vi "Main.vi"(8 "error in":errorcluster, 11 "Acq Cam Basler in":refnum<class "Acq Cam Basler.lvclass">) -> (0 "error out":errorcluster, 3 "Acq Cam Basler out":refnum<class "Acq Cam Basler.lvclass">)   [LabVIEW 2023, in "Acq Cam Basler.lvclass"]
doc: "The Queued Message Handler of a Worker."
uses:
  Acq Cam Basler.lvclass
  C:/Program Files (x86)/National Instruments/LabVIEW 2023/vi.lib/addons/_Workers/Library/Classes/Worker/Worker.lvclass
  Initialization Data.ctl
  UI Cam Basler/Parsed Data Acquisition.ctl
  UI Cam Basler/Data Image.ctl
  <vilib>/vision/Image Controls.llb/IMAQ Image.ctl
  <vilib>/addons/_Workers/Library/Classes/Message Queue/Message Queue.lvclass
  Etat Acquisition.ctl
  <vilib>/userDefined/High Color/IMAQdx.ctl
  Acq Cam Basler.lvclass/Acq Cam Basler.ctl
  <vilib>/addons/_Workers/Library/Classes/Message/Enqueue Message to Self v2 - Silent Mode.vi
  <vilib>/addons/_Workers/Library/Classes/Message/Message.lvclass
  <vilib>/vision/driver/NI_Vision_Acquisition_Software.lvlib
  UI Cam Basler/UI Cam Basler.lvclass
  C:/Program Files (x86)/National Instruments/LabVIEW 2023/vi.lib/addons/_Workers/Library/Classes/Workers Object/Workers Object.lvclass
  C:/Users/flepetit/Desktop/CamView-mdi-LV/Workers/Acq Cam Basler/Acq Cam Basler.lvclass
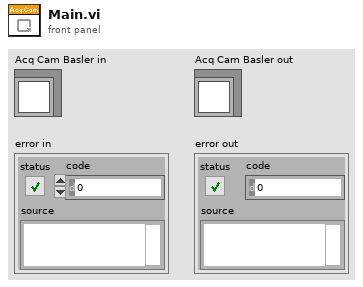
[diagram p1: front panel]
types:
  T1 = typedef "IMAQdx.ctl" = refnum<k21>
  T2 = typedef "Acq Cam Basler.lvclass/Etat Acquisition.ctl" = enum16{"Acquire", "Idle"}
  T3 = typedef "Acq Cam Basler.lvclass/Initialization Data.ctl" = cluster{"String":string, "Parsed Data Acquisition":T4, "Data Display":refnum<notifier>, "UI Cam Queue":refnum<class "Message Queue.lvclass">}
  T4 = typedef "UI Cam Basler.lvclass/Parsed Data Acquisition.ctl" = cluster{"Config Acquisition":cluster{"Camera name":string, "Gain":dbl, "Shutter(us)":dbl, "ROI":bool, "ROI coor":T5, "Palette":u32, "ModelName":string, "Pos X Ch":u32, "Pos Y Ch":u32, "Crosshair":bool}}
  T5 = typedef "IMAQ Rectangle" = cluster{"Left":i32, "Top":i32, "Right":i32, "Bottom":i32, "Rotation":dbl}
  T6 = typedef "IMAQ Image.ctl" = refnum<image>
  T7 = typedef "Workers.lvlib/Case Label.ctl" = string
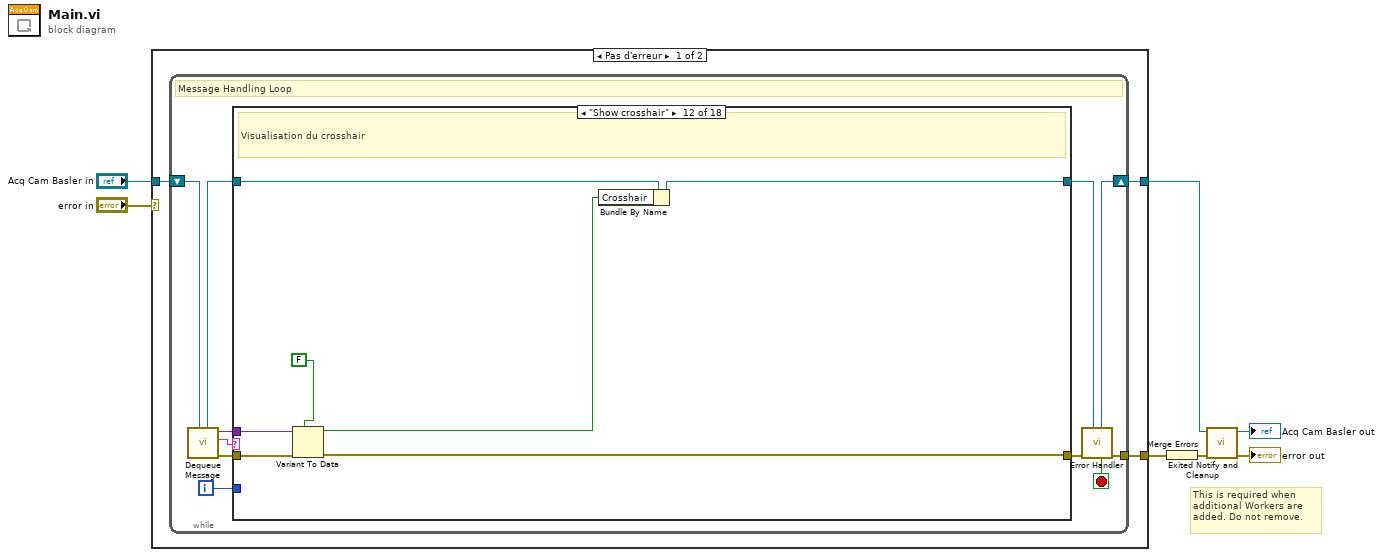
[diagram p0: block diagram]
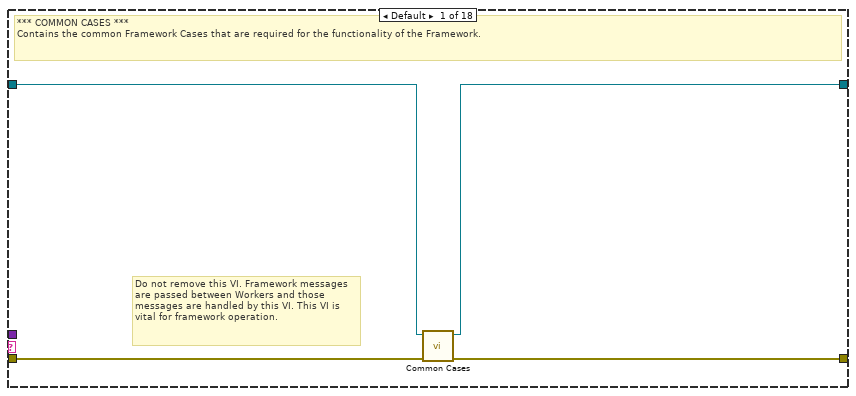
[diagram p2: hidden frame]
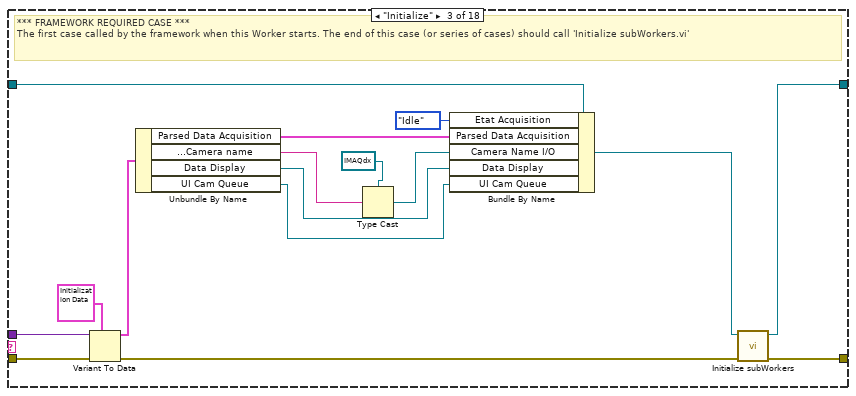
[diagram p4: hidden frame]
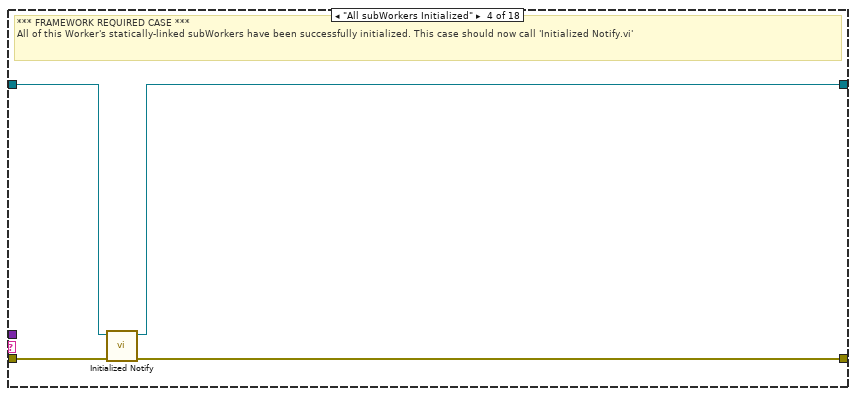
[diagram p5: hidden frame]
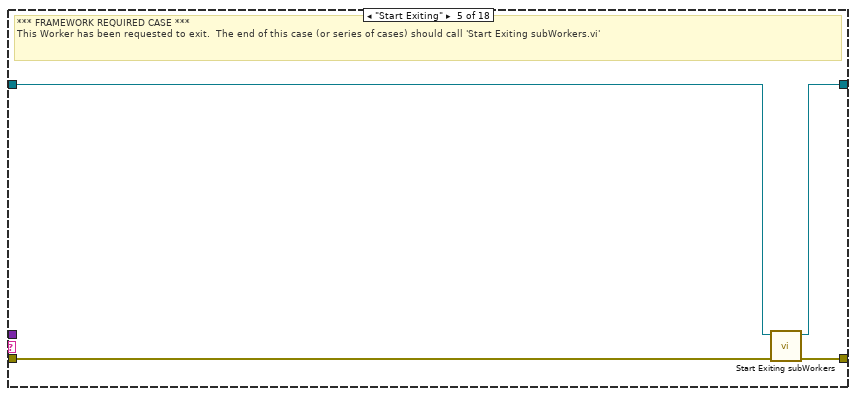
[diagram p6: hidden frame]
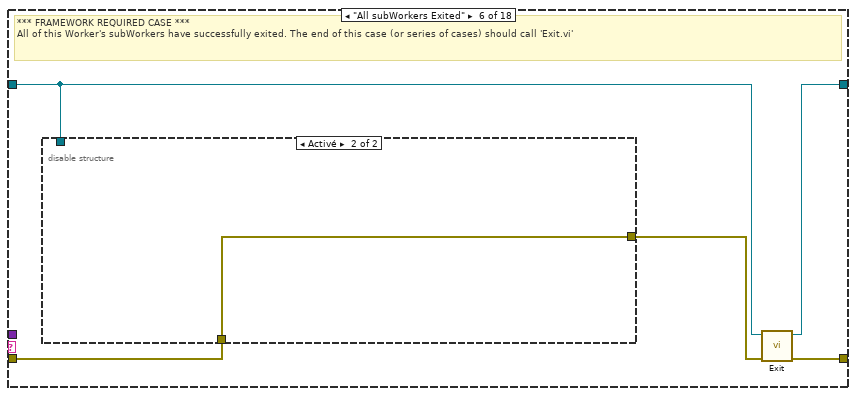
[diagram p7: hidden frame]
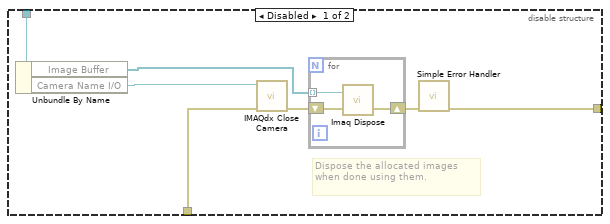
[diagram p8: hidden frame]
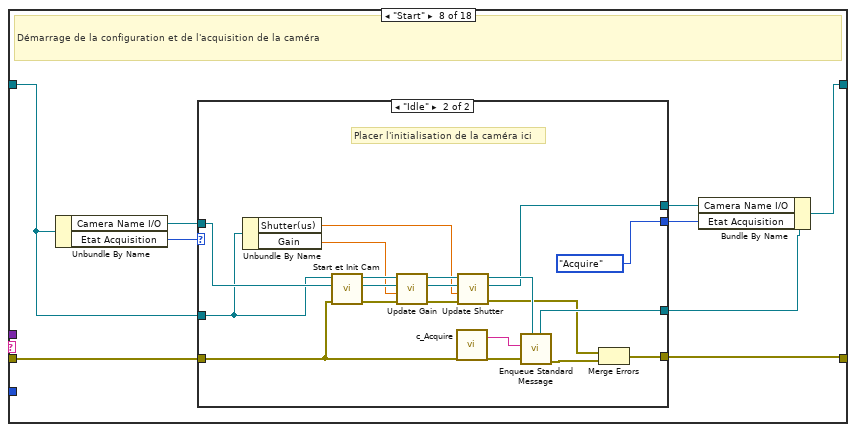
[diagram p10: hidden frame]
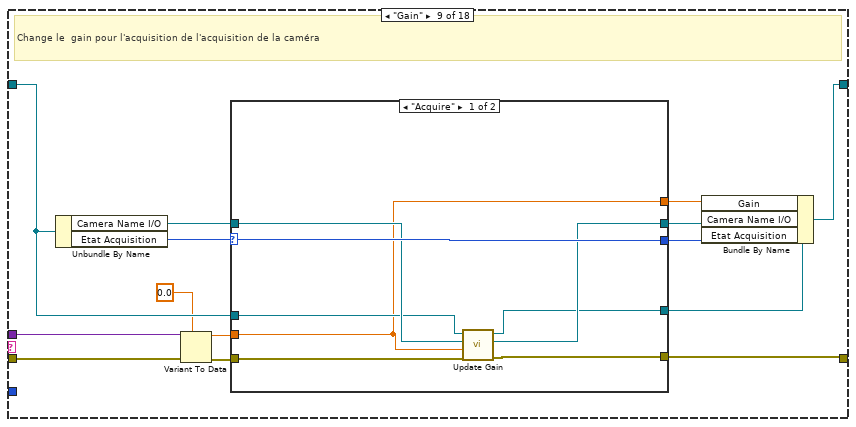
[diagram p12: hidden frame]
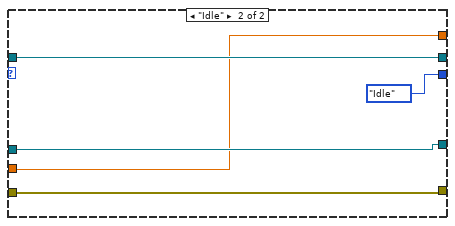
[diagram p13: hidden frame]
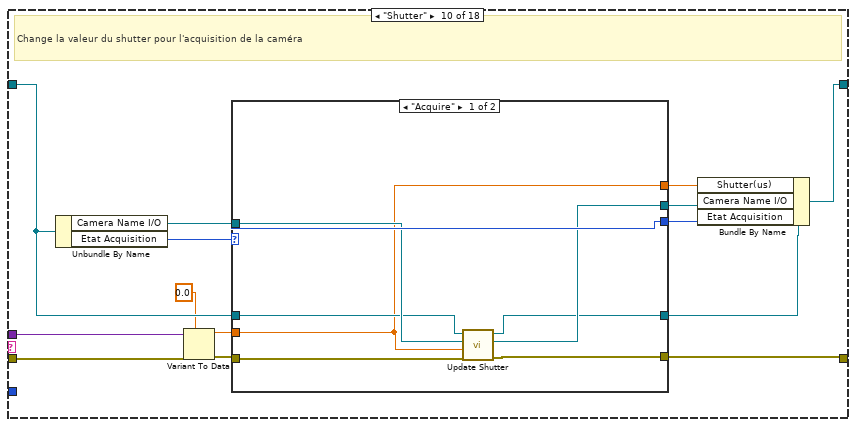
[diagram p14: hidden frame]
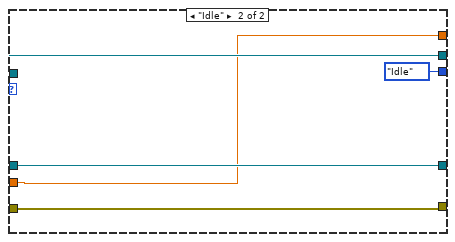
[diagram p15: hidden frame]
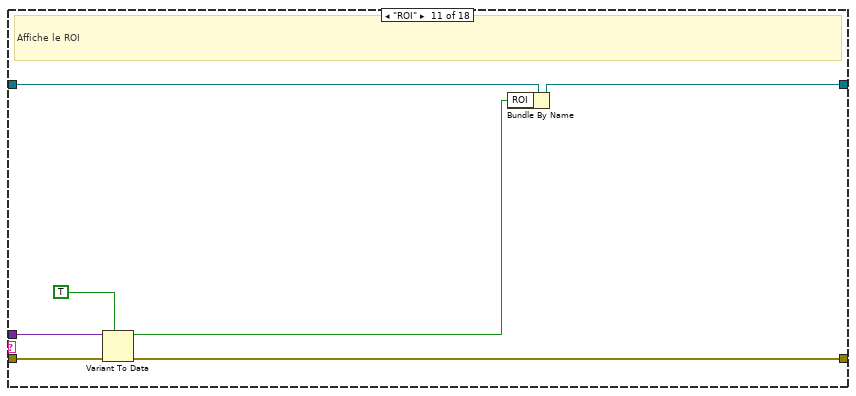
[diagram p16: hidden frame]
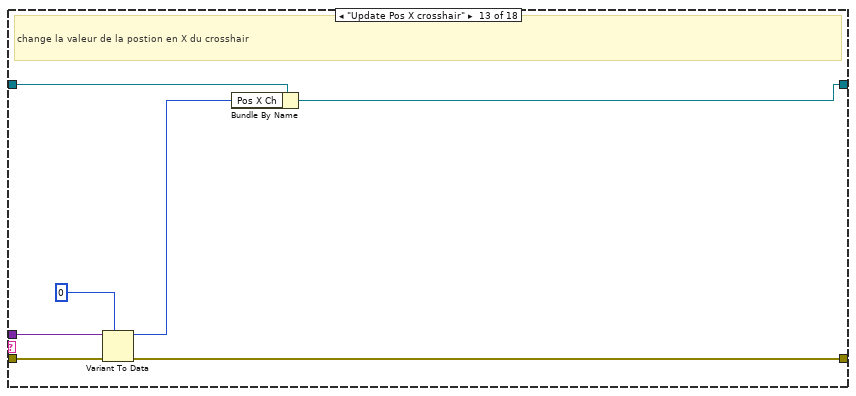
[diagram p17: hidden frame]
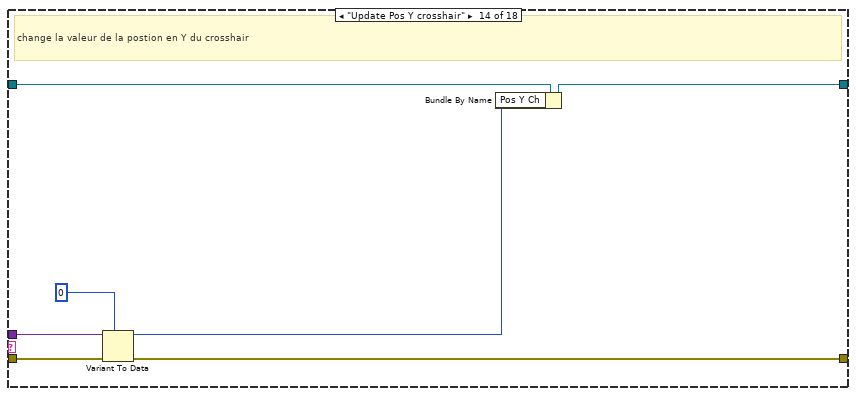
[diagram p18: hidden frame]
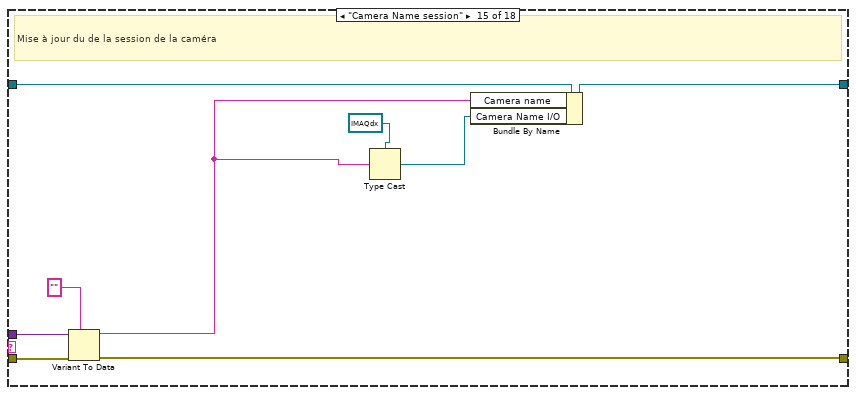
[diagram p19: hidden frame]
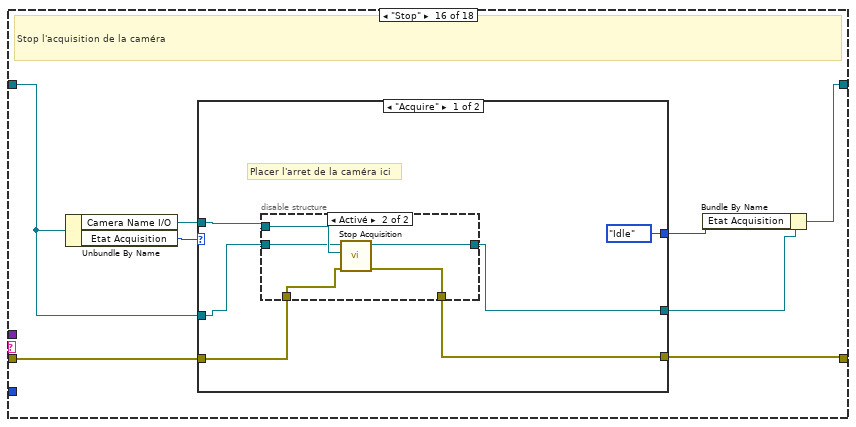
[diagram p20: hidden frame]
diagram:
  # "This is required when additional Workers are added. Do not remove."
  n1 = case shown="Pas d'erreur" "error in" {
    tunnel: "Acq Cam Basler in" -> [w8 w240]
    tunnel: [w10 w241] -> w6
    tunnel: [w9 w239] -> w7
    selector: "error in" -> [_ w242]
    frame No Error {
      n2 = while {
        shift-right: [w19] -> w9
        shift-left: w8 -> [w21]
        tunnel: [w20] -> w10
        i -> [w11]
        stop <- w12 stop-if-true
        # "Message Handling Loop"
        n3 = call-dynamic "Dequeue Message.vi"("Worker"=w21) -> ("error out"=w18:errorcluster, "Case out"=w13:string, "Data out"=w14:variant, "Worker out"=w16:refnum<class "Acq Cam Basler.lvclass">)  [unwired: 6 in, 1 out]
        n4 = case "Worker MHL Case Structure (DO NOT CHANGE LABEL NAME)" shown="\"Show crosshair\"" w13 {
          tunnel: w18 -> [w25 w26 w41 w47 w48 w54 w68 w75 w107 w133 w160 w168 w174 w181 w191 w197 w218 w222]
          tunnel: [w24 w26 w43 w46 w51 w56 w68 w74 w112 w139 w158 w166 w170 w179 w187 w196 w218 w221] -> w17
          tunnel: w16 -> [w23 w27 w40 w45 w49 w52 w69 w73 w111 w138 w161 w169 w175 w182 w192 w195 w219 w223]
          tunnel: [w22 w27 w42 w44 w50 w55 w69 w77 w114 w141 w157 w164 w171 w178 w189 w199 w219 w224] -> w15
          tunnel: w14 -> [_ _ w38 _ _ _ _ _ w105 w131 w159 w167 w173 w180 w190 _ _ _]
          tunnel: w11 -> [_ _ _ _ _ _ _ _ _ _ _ _ _ _ _ _ _ _]
          frame Default {
            # "Do not remove this VI. Framework messages are passed between Workers and those messages are handled by this VI. This VI is vital for framework operation."
            # "*** COMMON CASES ***\nContains the common Framework Cases that are required for the functionality of the Framework."
            n5 = call-dynamic "Common Cases.vi"("error in"=w25, "Worker in"=w23) -> ("error out"=w24:errorcluster, "Worker out"=w22:refnum<class "Acq Cam Basler.lvclass">)  [unwired: 8 in]
          }
          frame "------ FRAMEWORK REQUIRED CASES ------" {
            # "Start of Framework Required Cases"
          }
          frame "Initialize" {
            # "*** FRAMEWORK REQUIRED CASE ***\nThe first case called by the framework when this Worker starts. The end of this case (or series of cases) should call 'Initialize subWorkers.vi'"
            n6 = Variant To Data(error in=w41, type=T3 {"String"="", "Parsed Data Acquisition"={"Config Acquisition"={"Camera name"="", "Gain"=0.0, "Shutter(us)"=0.0, "ROI"=FALSE, "ROI coor"={"Left"=0, "Top"=0, "Right"=0, "Bottom"=0, "Rotation"=0.0}, "Palette"=5, "ModelName"="", "Pos X Ch"=0, "Pos Y Ch"=0, "Crosshair"=FALSE}}, "Data Display"=refnum, "UI Cam Queue"=refnum} ("Cluster"), Variant=w38) -> (data=w35:T3, error out=w39:errorcluster)
            n7 = Unbundle By Name(w35) -> ("Parsed Data Acquisition"=w34:T4, "Parsed Data Acquisition.Config Acquisition.Camera name"=w33:string, "Data Display"=w31:refnum<notifier>, "UI Cam Queue"=w28:refnum<class "Message Queue.lvclass">)
            n8 = Type Cast(type=T1 refnum ("Camera Name"), x=w33) -> (*(type *) &x=w30:T1)
            n9 = Bundle By Name(cluster=w40, "Etat Acquisition"=Etat_Acquisition."Idle", "Parsed Data Acquisition"=w34, "Camera Name I/O"=w30, "Data Display"=w31, "UI Cam Queue"=w28) -> (w29:refnum<class "Acq Cam Basler.lvclass">)
            n10 = call-dynamic "Initialize subWorkers.vi"("error in"=w39, "Worker"=w29) -> ("error out"=w43:errorcluster, "dup Worker out"=w42:refnum<class "Acq Cam Basler.lvclass">)  [unwired: 8 in]
          }
          frame "All subWorkers Initialized" {
            # "*** FRAMEWORK REQUIRED CASE ***\nAll of this Worker's statically-linked subWorkers have been successfully initialized. This case should now call 'Initialized Notify.vi'"
            n11 = call-dynamic "Initialized Notify.vi"("error in"=w47, "Worker"=w45) -> ("error out"=w46:errorcluster, "dup Worker out"=w44:refnum<class "Acq Cam Basler.lvclass">)  [unwired: 8 in]
          }
          frame "Start Exiting" {
            # "*** FRAMEWORK REQUIRED CASE ***\nThis Worker has been requested to exit.  The end of this case (or series of cases) should call 'Start Exiting subWorkers.vi'"
            n12 = call-dynamic "Start Exiting subWorkers.vi"("error_in"=w48, "Worker"=w49) -> ("error out"=w51:errorcluster, "dup Worker out"=w50:refnum<class "Acq Cam Basler.lvclass">)  [unwired: 8 in]
          }
          frame "All subWorkers Exited" {
            # "*** FRAMEWORK REQUIRED CASE ***\nAll of this Worker's subWorkers have successfully exited. The end of this case (or series of cases) should call 'Exit.vi'"
            n13 = disable-structure shown="Activé" {
              disable-tunnel: w54 -> [w61 w67]
              disable-tunnel: [w60 w67] -> w53
              disable-tunnel: w52 -> [w59 _]
              frame Disabled {
                # "Dispose the allocated images when done using them."
                n14 = Unbundle By Name(w59) -> ("Image Buffer"=w57:T6[], "Camera Name I/O"=w58:T1)
                n15 = call <vilib>:"IMAQdx Close Camera.vi"("error in"=w61, "Session In"=w58) -> ("error out"=w63:errorcluster)  [unwired: 9 out]
                n16 = for {
                  shift-right: [w65] -> w62
                  shift-left: w63 -> [w66]
                  tunnel: w57 -> [w64] mode=indexing
                  n17 = call "Imaq Dispose"("Image"=w64, "error in (no error)"=w66) -> ("error out"=w65:errorcluster)  [unwired: 4 in]
                }
                n18 = call <vilib>:"Simple Error Handler.vi"("error in (no error)"=w62) -> ("error out"=w60:errorcluster)  [unwired: 4 in, 4 out]
              }
              frame Enabled {
              }
            }
            n19 = call-dynamic "Exit.vi"("error_in"=w53, "Worker"=w52) -> ("error out"=w56:errorcluster, "dup Worker out"=w55:refnum<class "Acq Cam Basler.lvclass">)  [unwired: 8 in]
          }
          frame "-------------------From UI Cam Basler----------------------------" {
            # "End of Framework Required Cases"
          }
          frame "Start" {
            # "Démarrage de la configuration et de l'acquisition de la caméra"
            n20 = Unbundle By Name(w73) -> ("Camera Name I/O"=w71:T1, "Etat Acquisition"=w78:T2)
            n21 = case shown="\"Idle\"" w78 {
              selector: w78 -> [w82 _]
              tunnel: [w82 Etat_Acquisition."Acquire" ("Etat Acquisition")] -> w76
              tunnel: w75 -> [w80 w95]
              tunnel: [w80 w99] -> w74
              tunnel: w73 -> [w81 w85]
              tunnel: [w81 w97] -> w72
              tunnel: w71 -> [w79 w96]
              tunnel: [w79 w88] -> w70
              frame "Acquire" {
              }
              frame "Idle" {
                # "Placer l'initialisation de la caméra ici"
                n22 = Unbundle By Name(w85) -> ("Shutter(us)"=w83:dbl, "Gain"=w84:dbl)
                n23 = call "Start et Init Cam.vi"("error in (no error)"=w95, "Session In"=w96, "Acq Cam Basler en entrée"=w85) -> ("error out"=w92:errorcluster, "Session Out"=w94:T1, "Acq Cam Basler en sortie"=w93:refnum<class "Acq Cam Basler.lvclass">)  [unwired: 6 in]
                n24 = call "Update Gain.vi"("error in (no error)"=w92, "Gain"=w84, "IMAQdx Session in"=w94, "Acq Cam Basler en entrée"=w93) -> ("error out"=w91:errorcluster, "IMAQdx Session out"=w87:T1, "Acq Cam Basler en sortie"=w90:refnum<class "Acq Cam Basler.lvclass">)  [unwired: 5 in]
                n25 = call "c_Acquire.vi"() -> ("Case Label"=w98:T7)  [unwired: 1 in]
                n26 = call "Update Shutter.vi"("error in (no error)"=w91, "Shutter"=w83, "IMAQdx Session in"=w87, "Acq Cam Basler en entrée"=w90) -> ("error out"=w86:errorcluster, "IMAQdx Session out"=w88:T1, "Acq Cam Basler en sortie"=w89:refnum<class "Acq Cam Basler.lvclass">)  [unwired: 5 in]
                n27 = call-poly <vilib>:"Enqueue Standard Message.vi"("Worker"=w89, "error in"=w95, "Case Label"=w98) -> ("error out"=w100:errorcluster, "dup Worker out"=w97:refnum<class "Acq Cam Basler.lvclass">)  [unwired: 7 in]
                n28 = Merge Errors(w86, w100) -> (w99:errorcluster)
              }
            }
            n29 = Bundle By Name(cluster=w72, "Camera Name I/O"=w70, "Etat Acquisition"=w76) -> (w77:refnum<class "Acq Cam Basler.lvclass">)
          }
          frame "Gain" {
            # "Change le  gain pour l'acquisition de l'acquisition de la caméra"
            n30 = Unbundle By Name(w111) -> ("Camera Name I/O"=w109:T1, "Etat Acquisition"=w115:T2)
            n31 = Variant To Data(error in=w107, type=0.0, Variant=w105) -> (data=w104:dbl, error out=w106:errorcluster)
            n32 = case shown="\"Acquire\"" w115 {
              selector: w115 -> [w123 _]
              tunnel: [w123 Etat_Acquisition."Idle" ("Etat Acquisition")] -> w113
              tunnel: w106 -> [w117 w128]
              tunnel: [w118 w128] -> w112
              tunnel: w111 -> [w120 w126]
              tunnel: [w119 w126] -> w110
              tunnel: w109 -> [w122 w127]
              tunnel: [w121 w127] -> w108
              tunnel: w104 -> [w116 w124]
              tunnel: [w116 w124] -> w102
              frame "Acquire" {
                n33 = call "Update Gain.vi"("error in (no error)"=w117, "Gain"=w116, "IMAQdx Session in"=w122, "Acq Cam Basler en entrée"=w120) -> ("error out"=w118:errorcluster, "IMAQdx Session out"=w121:T1, "Acq Cam Basler en sortie"=w119:refnum<class "Acq Cam Basler.lvclass">)  [unwired: 5 in]
              }
              frame "Idle" {
              }
            }
            n34 = Bundle By Name(cluster=w110, "Gain"=w102, "Camera Name I/O"=w108, "Etat Acquisition"=w113) -> (w114:refnum<class "Acq Cam Basler.lvclass">)
          }
          frame "Shutter" {
            # "Change la valeur du shutter pour l'acquisition de la caméra"
            n35 = Unbundle By Name(w138) -> ("Camera Name I/O"=w136:T1, "Etat Acquisition"=w142:T2)
            n36 = Variant To Data(error in=w133, type=0.0, Variant=w131) -> (data=w130:dbl, error out=w132:errorcluster)
            n37 = case shown="\"Acquire\"" w142 {
              selector: w142 -> [w150 _]
              tunnel: [w150 Etat_Acquisition."Idle" ("Etat Acquisition")] -> w140
              tunnel: w132 -> [w144 w155]
              tunnel: [w145 w155] -> w139
              tunnel: w138 -> [w147 w153]
              tunnel: [w146 w153] -> w137
              tunnel: w136 -> [w149 w154]
              tunnel: [w148 w154] -> w135
              tunnel: w130 -> [w143 w151]
              tunnel: [w143 w151] -> w129
              frame "Acquire" {
                n38 = call "Update Shutter.vi"("error in (no error)"=w144, "Shutter"=w143, "IMAQdx Session in"=w149, "Acq Cam Basler en entrée"=w147) -> ("error out"=w145:errorcluster, "IMAQdx Session out"=w148:T1, "Acq Cam Basler en sortie"=w146:refnum<class "Acq Cam Basler.lvclass">)  [unwired: 5 in]
              }
              frame "Idle" {
              }
            }
            n39 = Bundle By Name(cluster=w137, "Shutter(us)"=w129, "Camera Name I/O"=w135, "Etat Acquisition"=w140) -> (w141:refnum<class "Acq Cam Basler.lvclass">)
          }
          frame "ROI" {
            # "Affiche le ROI"
            n40 = Variant To Data(error in=w160, type=TRUE, Variant=w159) -> (data=w156:bool, error out=w158:errorcluster)
            n41 = Bundle By Name(cluster=w161, "ROI"=w156) -> (w157:refnum<class "Acq Cam Basler.lvclass">)
          }
          frame "Show crosshair" {
            # "Visualisation du crosshair"
            n42 = Variant To Data(error in=w168, type=FALSE, Variant=w167) -> (data=w163:bool, error out=w166:errorcluster)
            n43 = Bundle By Name(cluster=w169, "Crosshair"=w163) -> (w164:refnum<class "Acq Cam Basler.lvclass">)
          }
          frame "Update Pos X crosshair" {
            # "change la valeur de la postion en X du crosshair"
            n44 = Variant To Data(error in=w174, type=u32 0, Variant=w173) -> (data=w172:u32, error out=w170:errorcluster)
            n45 = Bundle By Name(cluster=w175, "Pos X Ch"=w172) -> (w171:refnum<class "Acq Cam Basler.lvclass">)
          }
          frame "Update Pos Y crosshair" {
            # "change la valeur de la postion en Y du crosshair"
            n46 = Variant To Data(error in=w181, type=u32 0, Variant=w180) -> (data=w177:u32, error out=w179:errorcluster)
            n47 = Bundle By Name(cluster=w182, "Pos Y Ch"=w177) -> (w178:refnum<class "Acq Cam Basler.lvclass">)
          }
          frame "Camera Name session" {
            # "Mise à jour du de la session de la caméra"
            n48 = Variant To Data(error in=w191, type="", Variant=w190) -> (data=w185:string, error out=w187:errorcluster)
            n49 = Type Cast(type=T1 refnum ("Camera Name"), x=w185) -> (*(type *) &x=w184:T1)
            n50 = Bundle By Name(cluster=w192, "Camera name"=w185, "Camera Name I/O"=w184) -> (w189:refnum<class "Acq Cam Basler.lvclass">)
          }
          frame "Stop" {
            # "Stop l'acquisition de la caméra"
            n51 = Unbundle By Name(w195) -> ("Camera Name I/O"=w193:T1, "Etat Acquisition"=w200:T2)
            n52 = case shown="\"Acquire\"" w200 {
              selector: w200 -> [_ w215]
              tunnel: [Etat_Acquisition."Idle" ("Etat Acquisition") w215] -> w198
              tunnel: w197 -> [w205 w217]
              tunnel: [w204 w217] -> w196
              tunnel: w195 -> [w202 w216]
              tunnel: [w201 w216] -> w194
              tunnel: w193 -> [w203 _]
              frame "Acquire" {
                # "Placer l'arret de la caméra ici"
                n53 = disable-structure shown="Activé" {
                  disable-tunnel: w205 -> [w209 w212]
                  disable-tunnel: [w207 w211] -> w204
                  disable-tunnel: w203 -> [_ w214]
                  disable-tunnel: w202 -> [_ w213]
                  disable-tunnel: [_ w210] -> w201
                  frame Disabled {
                    n54 = call <vilib>:"IMAQdx Stop Acquisition.vi"("error in"=w209) -> ("error out"=w208:errorcluster)  [unwired: 9 in, 1 out]
                    n55 = call <vilib>:"IMAQdx Close Camera.vi"("error in"=w208) -> ("error out"=w207:errorcluster)  [unwired: 10 in]
                  }
                  frame Enabled {
                    n56 = call "Stop Acquisition.vi"("error in (no error)"=w212, "Session In"=w214, "Acq Cam Basler en entrée"=w213) -> ("error out"=w211:errorcluster, "Acq Cam Basler en sortie"=w210:refnum<class "Acq Cam Basler.lvclass">)  [unwired: 7 in]
                  }
                }
              }
              frame "Idle" {
              }
            }
            n57 = Bundle By Name(cluster=w194, "Etat Acquisition"=w198) -> (w199:refnum<class "Acq Cam Basler.lvclass">)
          }
          frame "--------------------------------Himself-------------------------------" {
            # "End of Framework Required Cases"
          }
          frame "Acquire" {
            # "Démarrage de la configuration et de l'acquisition de la caméra"
            n58 = Unbundle By Name(w223) -> ("Camera Name I/O"=w220:T1, "Etat Acquisition"=w225:T2)
            n59 = case shown="\"Acquire\"" w225 {
              tunnel: [w234 w238] -> w224
              tunnel: w223 -> [w229 w238]
              tunnel: w222 -> [w232 w237]
              tunnel: [w235 w237] -> w221
              tunnel: w220 -> [w230 _]
              frame "Acquire" {
                n60 = call "Acquisition.vi"("error in (no error)"=w232, "Session In"=w230, "Acq Cam Basler en entrée"=w229) -> ("error out"=w231:errorcluster, "Session Out"=w226:T1, "Acq Cam Basler en sortie"=w228:refnum<class "Acq Cam Basler.lvclass">)  [unwired: 6 in]
                n61 = Bundle By Name(cluster=w228, "Camera Name I/O"=w226) -> (w227:refnum<class "Acq Cam Basler.lvclass">)
                n62 = call "c_Acquire.vi"() -> ("Case Label"=w233:T7)  [unwired: 1 in]
                n63 = call-poly <vilib>:"Enqueue Standard Message.vi"("Worker"=w227, "error in"=w232, "Case Label"=w233) -> ("error out"=w236:errorcluster, "dup Worker out"=w234:refnum<class "Acq Cam Basler.lvclass">)  [unwired: 7 in]
                n64 = Merge Errors(w231, w236) -> (w235:errorcluster)
              }
              frame "Idle" {
              }
            }
          }
        }
        n65 = call-dynamic "Error Handler.vi"("Worker"=w15, "error_in"=w17) -> ("error out"=w20:errorcluster, "Stop Loop"=w12:bool, "Worker out"=w19:refnum<class "Acq Cam Basler.lvclass">)  [unwired: 7 in]
      }
    }
    frame Error {
      n66 = call-dynamic "Error Handler.vi"("Worker"=w240, "error_in"=w242) -> ("error out"=w241:errorcluster, "Worker out"=w239:refnum<class "Acq Cam Basler.lvclass">)  [unwired: 7 in, 1 out]
    }
  }
  n67 = Merge Errors(w6) -> (w3:errorcluster)
  n68 = call-dynamic "Exited Notify and Cleanup.vi"("error_in"=w3, "Worker"=w7) -> ("error out"=→"error out":errorcluster, "dup Worker out"=→"Acq Cam Basler out":refnum<class "Acq Cam Basler.lvclass">)  [unwired: 8 in]
